vi "ChangeFlowrate.vi"(0 "Flowrate":dbl, 2 "Serial Port in":refnum<visa-resource-name>) -> (1 "error out":errorcluster)   [LabVIEW 2018]
uses:
  <instrlib>/Chemyx/_driver/Basic driver/Communication/controls/comm_rate_enum.ctl
  <instrlib>/Chemyx/_driver/Chemyx_Syringe_Pump_driver.lvlib
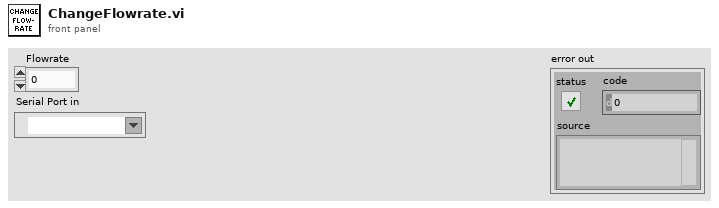
[diagram p1: front panel]
types:
  T1 = typedef "Chemyx_Syringe_Pump_driver.lvlib/comm_rate_enum.ctl" = enum16{"9600", "38400"}
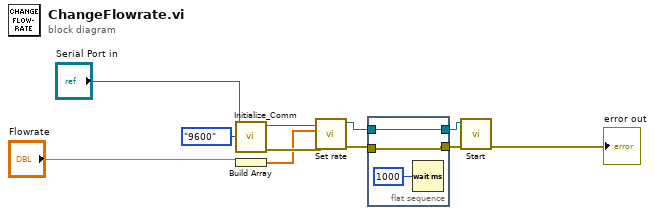
[diagram p0: block diagram]
diagram:
  n1 = call <instrlib>:"Initialize_Comm.vi"("Baud rate"=comm_rate_enum."9600", "Serial Port in"="Serial Port in") -> ("error out"=w11:errorcluster, "Serial Port out"=w10:refnum<visa-resource-name>)  [unwired: 8 in]
  n2 = Build Array("Flowrate") -> (w9:dbl[])
  n3 = call <instrlib>:"Set rate.vi"("error in (no error)"=w11, "Rate (array)"=w9, "Serial Port in"=w10) -> ("error out"=w4:errorcluster, "Serial Port out"=w7:refnum<visa-resource-name>)  [unwired: 7 in]
  n4 = flat-sequence {
    tunnel: w7 -> [w14]
    tunnel: [w14] -> w6
    tunnel: w4 -> [w13]
    tunnel: [w13] -> w5
    frame #0 {
      n5 = Wait (ms)(milliseconds to wait=u32 1000) -> ()  [unwired: 1 out]
    }
  }
  n6 = call <instrlib>:"Start.vi"("error in (no error)"=w5, "Serial Port in"=w6) -> ("error out"=→"error out":errorcluster)  [unwired: 8 in, 1 out]
